vi "Remove Routing Channel.vi"(8 "error in":errorcluster, 10 "routing channel name":string, 11 "routing channels in":T1 format="%.0x") -> (0 "error out":errorcluster, 3 "routing channels out":T1 format="%.0x")   [LabVIEW 2017, in "Routing and Faulting Scripting.lvlib"]
uses:
  Routing and Faulting Scripting.lvlib
  <vilib>/NI Veristand/Custom Device API/Custom Device Item Ref.ctl
  <vilib>/NI Veristand/Custom Device API/Custom Device API.lvlib
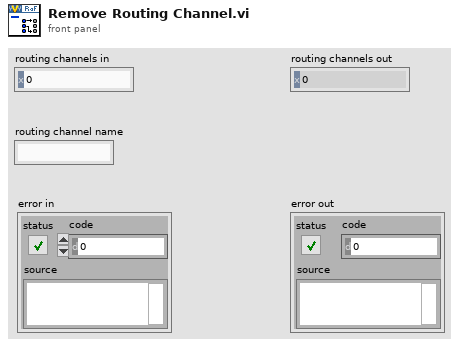
[diagram p1: front panel]
types:
  T1 = typedef "Custom Device API.lvlib/Custom Device Item Ref.ctl" = u64
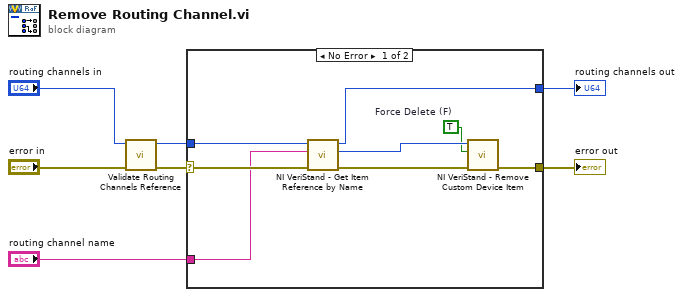
[diagram p0: block diagram]
diagram:
  n1 = call "Validate Routing Channels Reference.vi"("error in"="error in", "routing channels in"="routing channels in") -> ("error out"=w3:errorcluster, "routing channels out"=w1:T1)  [unwired: 8 in]
  n2 = case shown="No Error" w3 {
    selector: w3 -> [w14 w17]
    tunnel: [w8 w17] -> w7
    tunnel: [w11 w16] -> w6
    tunnel: w1 -> [w15 w16]
    tunnel: "routing channel name" -> [w13 _]
    frame No Error {
      w9 = TRUE  # Force Delete (F)
      n3 = call <vilib>:"NI VeriStand - Get Item Reference by Name.vi"("error in (no error)"=w14, "Item Name"=w13, "Parent Ref in"=w15) -> ("error out"=w10:errorcluster, "Item Ref"=w12:T1, "Parent Ref out"=w11:T1)  [unwired: 5 in, 1 out]
      n4 = call <vilib>:"NI VeriStand - Remove Custom Device Item.vi"("error in (no error)"=w10, "Force Delete (F)"=w9, "Item Ref in"=w12) -> ("error out"=w8:errorcluster)  [unwired: 7 in, 1 out]
    }
    frame Error {
    }
  }
  "error out" <- w7
  "routing channels out" <- w6
